vi "pdtV4Main.vi"() -> ()   [LabVIEW 2021]
uses:
  <vilib>/DAQmx/read.llb/DAQmx Read (Analog 1D DBL NChan 1Samp).vi
  <vilib>/DAQmx/create/channels.llb/DAQmx Create Channel (AI-Voltage-Basic).vi
  <vilib>/DAQmx/configure/timing.llb/DAQmx Timing (Sample Clock).vi
  <vilib>/Utility/file.llb/Read Delimited Spreadsheet (DBL).vi
  <vilib>/DAQmx/miscellaneous.llb/DAQmx Fill In Error Info.vi
panel:
  in  "Test time / ms":u32=10000
  out "Pitch y":dbl
  in  "Emergency Stop":bool
  in  "Idle pos":bool
  out "Pitch x":dbl
  in  "Group\nQuantity Y":i32=1
  in  "Group\nQuantity X":i32=1
  out "Initial Y":dbl
  out "Initnal X":dbl
  in  "ConfirmCrd":bool
  out "Instruction":string
  in  "New plate":bool
  in  "Timed Run":bool
  in  "Fine Adjust":bool
  in  "Crd Zero":bool
  out "y":dbl
  out "x":dbl
  in  "Right":bool
  in  "Down":bool
  in  "Left":bool
  in  "Up":bool
  in  "pwm level / 20":i32
  in  "Power Calibration / mW":dbl
  in  "Manual Coordinate Adjustment":bool
  in  "Start PDT":bool
  in  "Plate type":i32(ring) items=["single cell", "96-well 3x3", "96-well 3x2 (horizontal)", "96-well 2x3 (vertical)", "96-well ULA 3x3", "96-well ULA LND 3x2", "24-well 2x2", "96-well flat bottom 3x3 good one"]
  in  "Plate dose / J cm2":dbl[][](array[numeric])
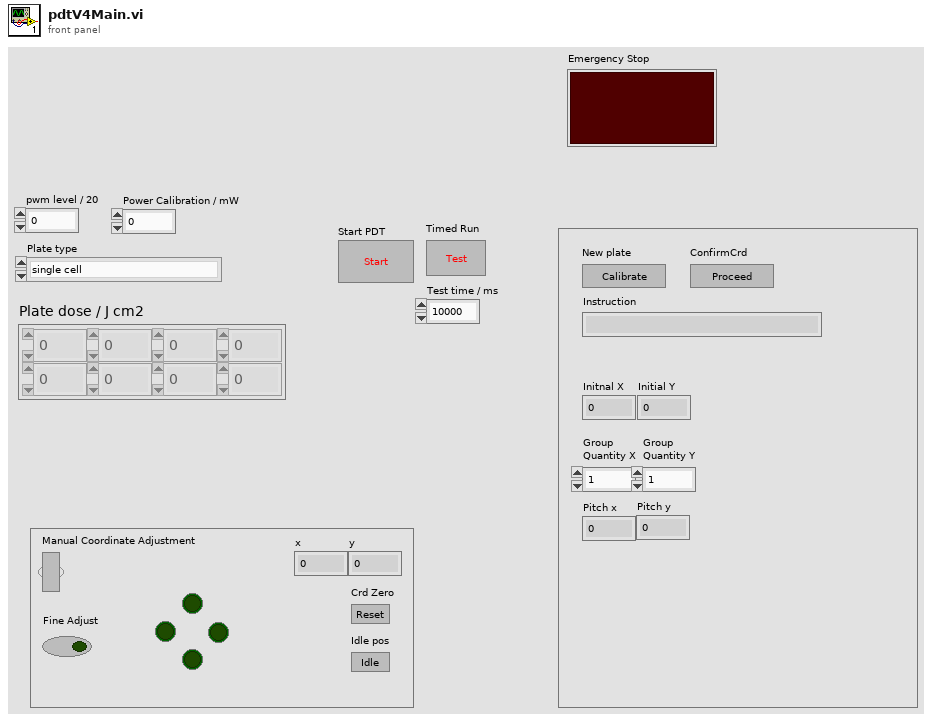
[diagram p1: front panel]
types:
  T1 = enum8{"Enabled", "Disabled", "Disabled and Grayed Out"}
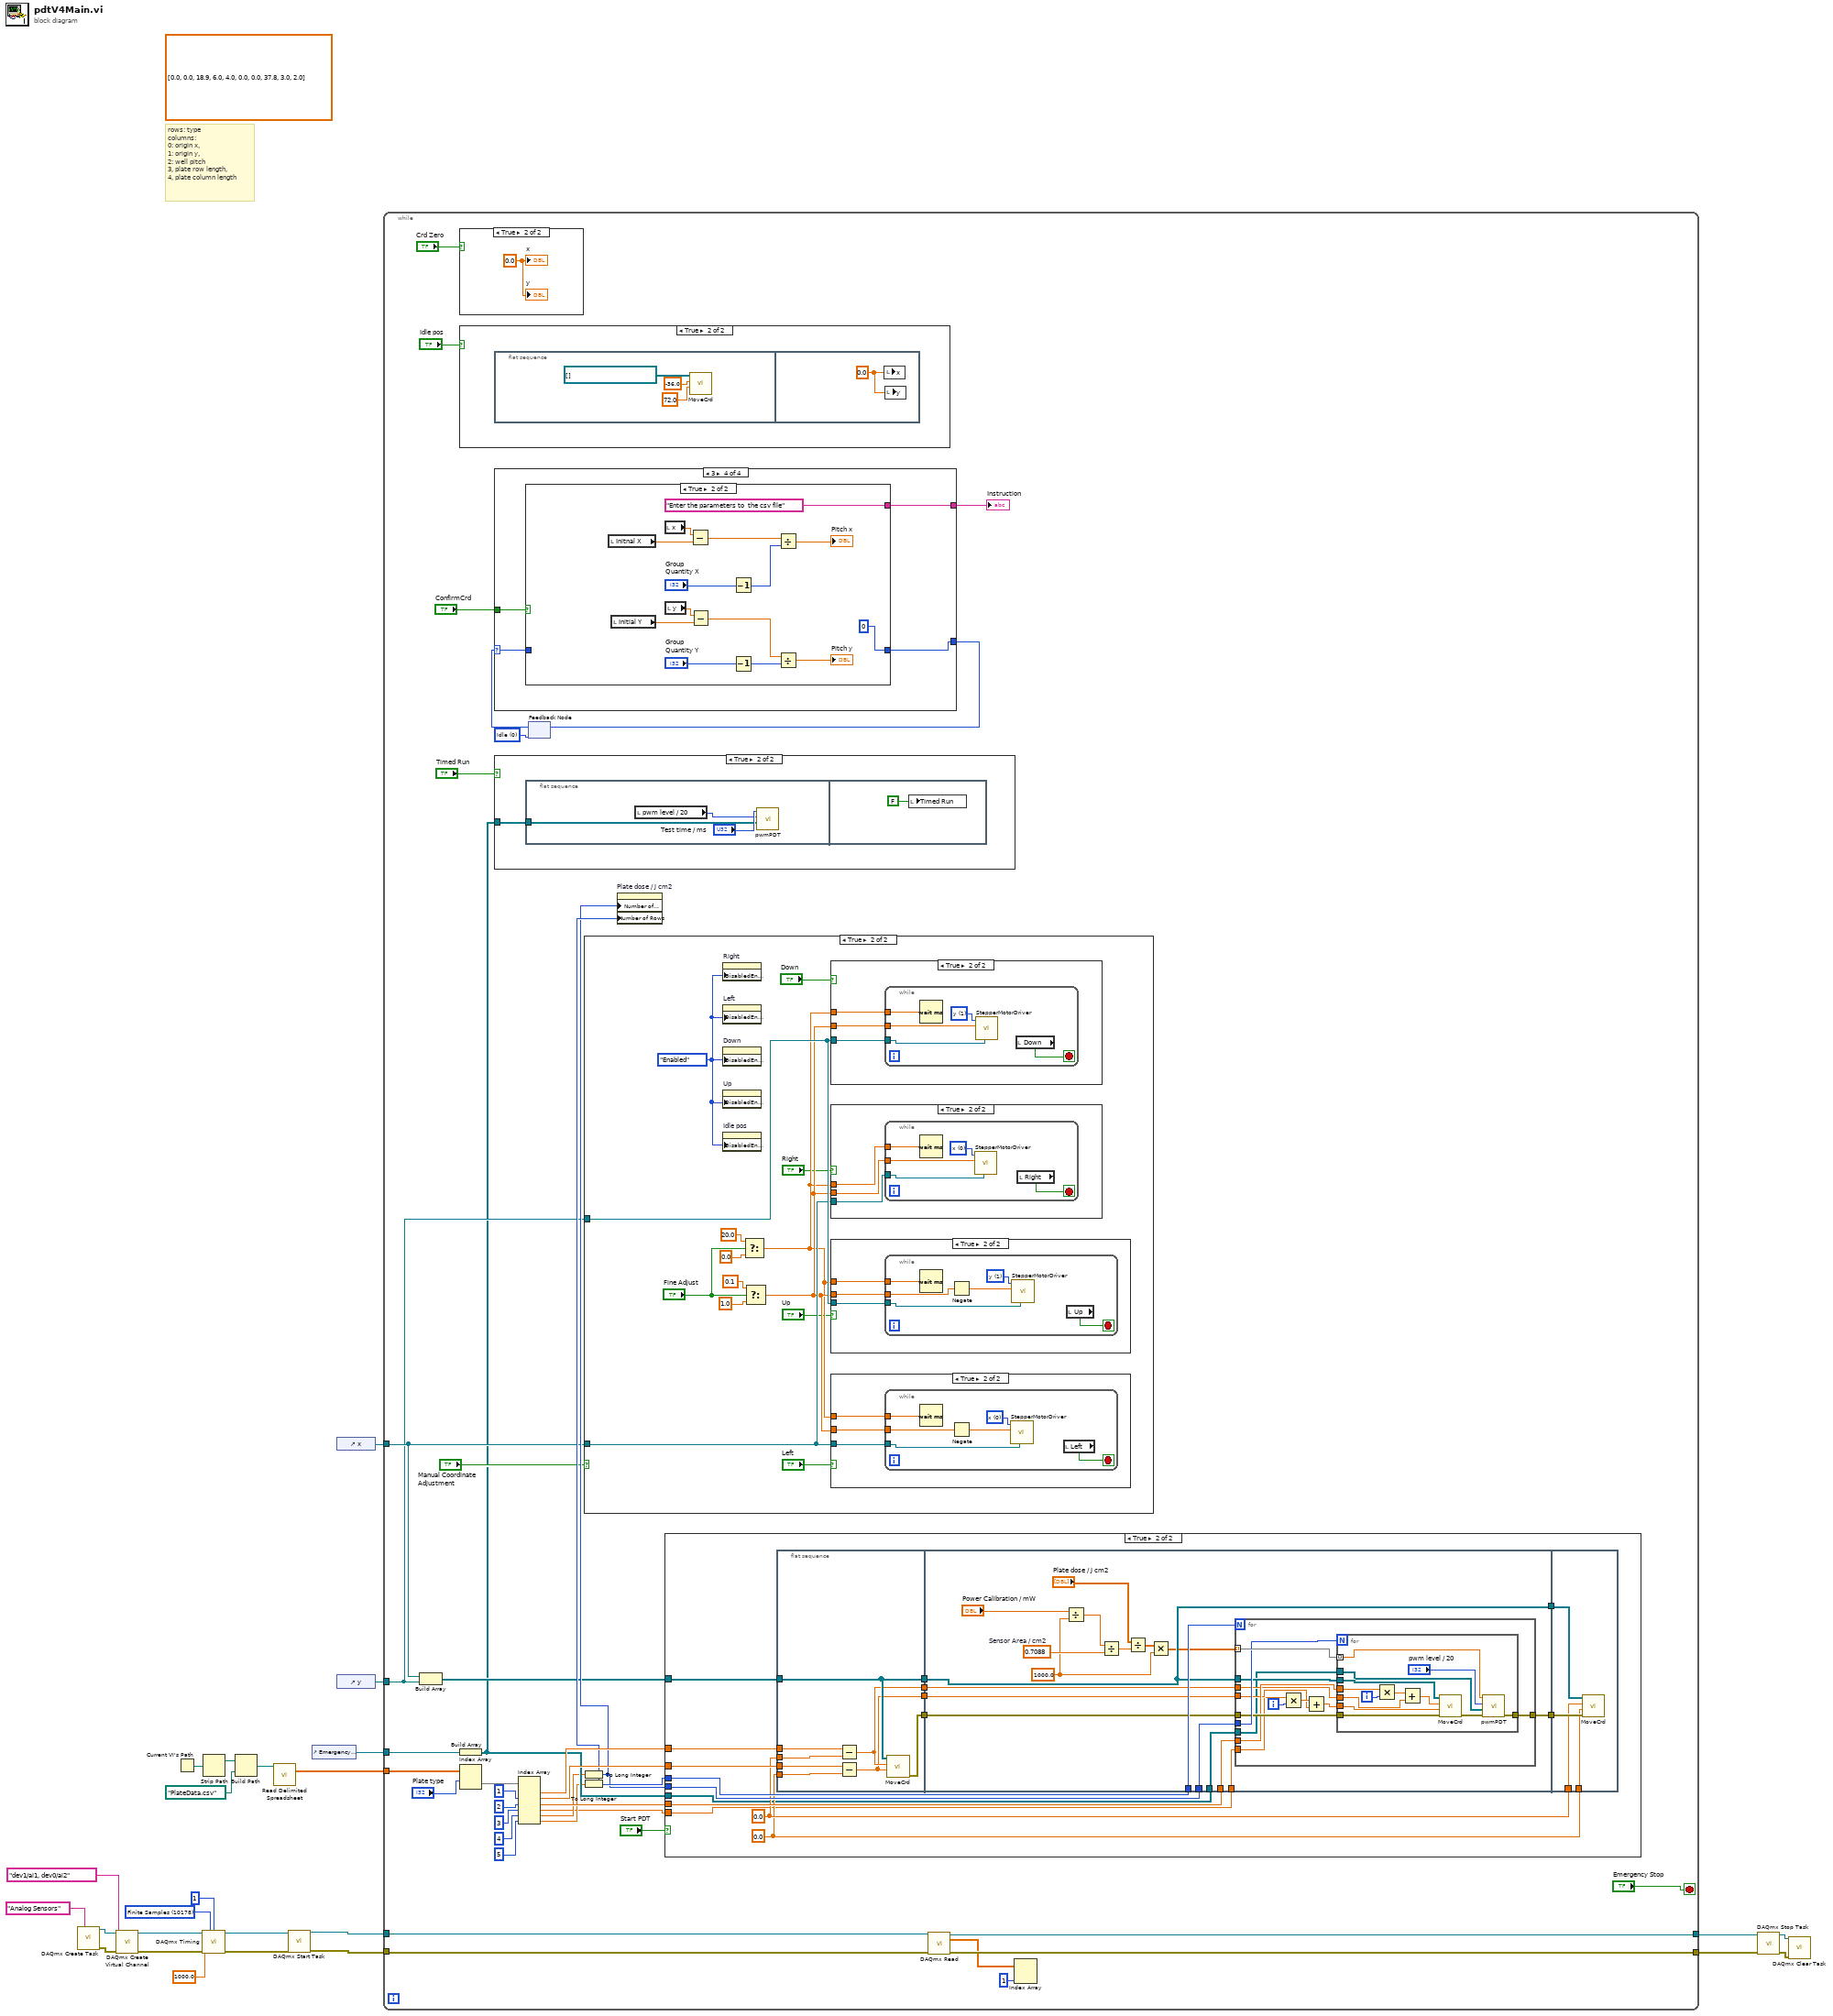
[diagram p0: block diagram]
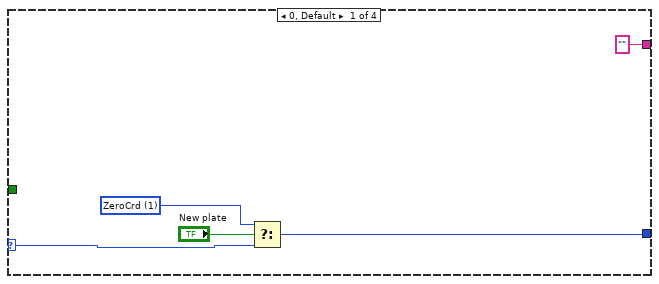
[diagram p3: hidden frame]
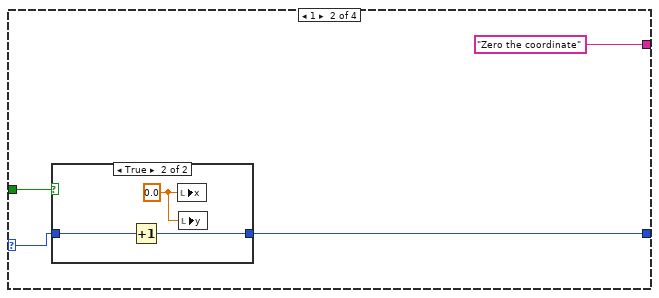
[diagram p4: hidden frame]
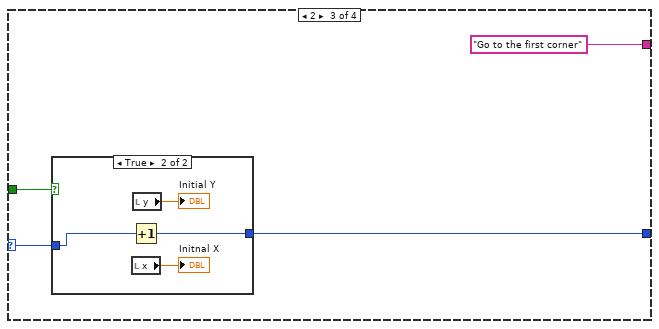
[diagram p6: hidden frame]
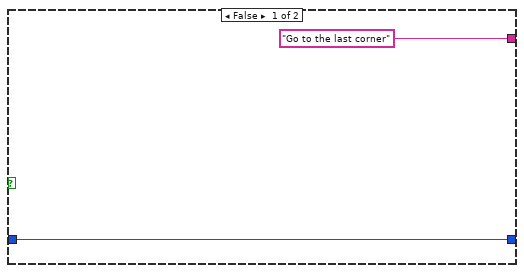
[diagram p8: hidden frame]
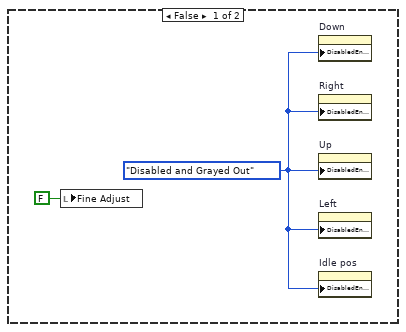
[diagram p11: hidden frame]
diagram:
  w3 = 10178 items=["Finite Samples"=10178, "Continuous Samples"=10123, "Hardware Timed Single Point"=12522] ("sample mode")
  (unwired) dbl[][] [[0.0, 0.0, 18.9, 6.0, 4.0], [0.0, 0.0, 37.8, 3.0, 2.0]]
  # "rows: type\ncolumns: \n0: origin x, \n1: origin y, \n2: well pitch\n3, plate row length, \n4, plate column length"
  n1 = call <vilib>:"DAQmx Create Task.vi"("new task name"="Analog Sensors") -> ("task out"=w7:refnum<k21>, "error out"=w6:errorcluster)  [unwired: 13 in]
  n2 = call-poly <vilib>:"DAQmx Create Virtual Channel.vi"("task in"=w7, "physical channels"=tag "dev1/ai1, dev0/ai2", "error in"=w6) -> ("task out"=w17:refnum<k21>, "error out"=w16:errorcluster)  [unwired: 11 in]
  n3 = Current VI's Path() -> (path=w22:path)
  n4 = call-poly <vilib>:"DAQmx Timing.vi"("task/channels in"=w17, "sample mode"=w3, "samples per channel"=1, "rate"=1000.0, "error in"=w16) -> ("task out"=w15:refnum<k21>, "error out"=w14:errorcluster)  [unwired: 9 in]
  n5 = Strip Path(path=w22) -> (stripped path=w21:path)  [unwired: 1 out]
  n6 = Build Path(base path=w21, name or relative path=path "PlateData.csv" ("file path (dialog if empty)")) -> (appended path=w24:path)
  n7 = call-poly <vilib>:"Read Delimited Spreadsheet.vi"("file path (dialog if empty)"=w24) -> ("all rows"=w25:dbl[][])  [unwired: 9 in, 5 out]
  n8 = call <vilib>:"DAQmx Start Task.vi"("task/channels in"=w15, "error in"=w14) -> ("task out"=w13:refnum<k21>, "error out"=w12:errorcluster)  [unwired: 12 in]
  n9 = control-ref of="Emergency Stop"() -> (w18:refnum<vi>)
  n10 = control-ref of="x"() -> (w20:refnum<vi>)
  n11 = control-ref of="y"() -> (w19:refnum<vi>)
  n12 = while {
    tunnel: w25 -> [w59]
    tunnel: w20 -> [w48]
    tunnel: w19 -> [w40]
    tunnel: w18 -> [w37]
    tunnel: w13 -> [w31]
    tunnel: w12 -> [w30]
    tunnel: [w29] -> w11
    tunnel: [w28] -> w10
    stop <- "Emergency Stop" stop-if-true
    w44 = u16 0 items=["Idle", "ZeroCrd", "StartCorner", "EndCorner"]
    n13 = Build Array(w48, w40) -> (w49:refnum<vi>[])
    n14 = case shown="True" "Crd Zero" {
      frame False {
      }
      frame True {
        w115 = 0.0 ("x")
        "x" <- w115
        "y" <- w115
      }
    }
    n15 = case shown="True" "Idle pos" {
      frame False {
      }
      frame True {
        n16 = flat-sequence {
          frame #0 {
            n17 = call "MoveCrd.vi"("FinalY"=72.0, "FinalX"=-36.0, "Current Crd"=refnum<vi>[] []) -> ()  [unwired: 8 in, 1 out]
          }
          frame #1 {
            w67 = 0.0
            n18 = local write "x"(w67) -> ()
            n19 = local write "y"(w67) -> ()
          }
        }
      }
    }
    n20 = Build Array(w37) -> (w36:refnum<vi>[])
    n21 = Index Array(array=w59, index (row)="Plate type") -> (element=w63:dbl[])  [unwired: 1 in]
    n22 = case shown="True" "Timed Run" {
      tunnel: w36 -> [_ w110]
      frame False {
      }
      frame True {
        n23 = flat-sequence {
          tunnel: w110 -> [w111]
          frame #0 {
            n24 = local read "pwm level / 20"() -> (w112:i32)
            n25 = call "pwmPDT.vi"("EmergencyStop"=w111, "pwm level / 20"=w112, "SetTime / ms"="Test time / ms") -> ()  [unwired: 8 in, 1 out]
          }
          frame #1 {
            n26 = local write "Timed Run"(FALSE ("10 sec pwm")) -> ()
          }
        }
      }
    }
    n27 = Index Array(array=w63, index #2=1 ("index"), index #3=2 ("index"), index #4=3 ("index"), index #5=4 ("index"), index #6=5 ("index")) -> (element #1=w55:dbl, element #2=w54:dbl, element #3=w51:dbl, element #4=w32:dbl, element #5=w33:dbl, element #6=w34:dbl)  [unwired: 1 in]
    n28 = feedback #1(w44) -> (w45:u16)
    n29 = case shown="3" w45 {
      selector: w45 -> [w69 w75 w81 w91]
      tunnel: [w71 w74 w82 w92] -> w43
      tunnel: "ConfirmCrd" -> [_ w76 w83 w93]
      tunnel: ["" ("String") "Zero the coordinate" ("String") "Go to the first corner" ("String") w90] -> w41
      frame 0, Default {
        w72 = u16 1 items=["Idle", "ZeroCrd", "StartCorner", "EndCorner"]
        n30 = Select(t=w72, s="New plate", f=w69) -> (s? t:f=w71:u16)
      }
      frame 1 {
        n31 = case shown="True" w76 {
          tunnel: w75 -> [w77 w79]
          tunnel: [w77 w78] -> w74
          frame False {
          }
          frame True {
            w80 = 0.0
            n32 = Increment(x=w79) -> (x+1=w78:u16)
            n33 = local write "x"(w80) -> ()
            n34 = local write "y"(w80) -> ()
          }
        }
      }
      frame 2 {
        n35 = case shown="True" w83 {
          tunnel: w81 -> [w85 w89]
          tunnel: [w85 w88] -> w82
          frame False {
          }
          frame True {
            n36 = Increment(x=w89) -> (x+1=w88:u16)
            n37 = local read "x"() -> (→"Initnal X":dbl)
            n38 = local read "y"() -> (→"Initial Y":dbl)
          }
        }
      }
      frame 3 {
        n39 = case shown="True" w93 {
          tunnel: [w95 u16 0] -> w92
          tunnel: w91 -> [w95 _]
          tunnel: ["Go to the last corner" ("String") "Enter the parameters to  the csv file" ("String")] -> w90
          frame False {
          }
          frame True {
            n40 = local read "Initnal X"() -> (w108:dbl)
            n41 = local read "Initial Y"() -> (w105:dbl)
            n42 = local read "x"() -> (w109:dbl)
            n43 = local read "y"() -> (w106:dbl)
            n44 = Subtract(x=w109, y=w108) -> (x-y=w107:dbl)
            n45 = Subtract(x=w106, y=w105) -> (x-y=w104:dbl)
            n46 = Decrement(x="Group\nQuantity X") -> (x-1=w101:i32)
            n47 = Decrement(x="Group\nQuantity Y") -> (x-1=w99:i32)
            n48 = Divide(x=w107, y=w101) -> (x/y=→"Pitch x":dbl)
            n49 = Divide(x=w104, y=w99) -> (x/y=→"Pitch y":dbl)
          }
        }
      }
    }
    "Instruction" <- w41
    n50 = feedback-in #1(w43) -> ()
    n51 = To Long Integer(number=w33) -> (32bit integer=w52:i32)
    n52 = To Long Integer(number=w34) -> (32bit integer=w53:i32)
    n53 = case shown="True" "Manual Coordinate Adjustment" {
      tunnel: w40 -> [_ w131]
      tunnel: w48 -> [_ w130]
      frame False {
        w116 = T1."Disabled and Grayed Out" ("Disabled")
        n54 = local write "Fine Adjust"(FALSE ("Fine Adjust")) -> ()
        n55 = property on="Down" class="Bool (strict)"("DisabledEnum"=w116) -> ()  [unwired: 2 in, 2 out]
        n56 = property on="Right" class="Bool (strict)"("DisabledEnum"=w116) -> ()  [unwired: 2 in, 2 out]
        n57 = property on="Up" class="Bool (strict)"("DisabledEnum"=w116) -> ()  [unwired: 2 in, 2 out]
        n58 = property on="Left" class="Bool (strict)"("DisabledEnum"=w116) -> ()  [unwired: 2 in, 2 out]
        n59 = property on="Idle pos" class="Bool"("DisabledEnum"=w116) -> ()  [unwired: 2 in, 2 out]
      }
      frame True {
        w118 = T1."Enabled" ("Disabled")
        n60 = property on="Right" class="Bool (strict)"("DisabledEnum"=w118) -> ()  [unwired: 2 in, 2 out]
        n61 = property on="Left" class="Bool (strict)"("DisabledEnum"=w118) -> ()  [unwired: 2 in, 2 out]
        n62 = property on="Down" class="Bool (strict)"("DisabledEnum"=w118) -> ()  [unwired: 2 in, 2 out]
        n63 = property on="Up" class="Bool (strict)"("DisabledEnum"=w118) -> ()  [unwired: 2 in, 2 out]
        n64 = property on="Idle pos" class="Bool"("DisabledEnum"=w118) -> ()  [unwired: 2 in, 2 out]
        n65 = Select(t=20.0, s="Fine Adjust", f=0.0) -> (s? t:f=w123:dbl)
        n66 = Select(t=0.1, s="Fine Adjust", f=1.0) -> (s? t:f=w127:dbl)
        n67 = case shown="True" "Down" {
          tunnel: w131 -> [_ w134]
          tunnel: w127 -> [_ w133]
          tunnel: w123 -> [_ w132]
          frame False {
          }
          frame True {
            n68 = while {
              tunnel: w134 -> [w137]
              tunnel: w133 -> [w136]
              tunnel: w132 -> [w135]
              stop <- w138 stop-if-true
              w139 = u16 1 items=["x", "y"] ("Direction")
              n69 = Wait (ms)(milliseconds to wait=w135) -> ()  [unwired: 1 out]
              n70 = call "StepperMotorDriver.vi"("pCoordinate"=w137, "Distance"=w136, "Direction"=w139) -> ()  [unwired: 8 in, 1 out]
              n71 = local read "Down"() -> (w138:bool)
            }
          }
        }
        n72 = case shown="True" "Right" {
          tunnel: w130 -> [_ w151]
          tunnel: w127 -> [_ w150]
          tunnel: w123 -> [_ w149]
          frame False {
          }
          frame True {
            n73 = while {
              tunnel: w151 -> [w154]
              tunnel: w150 -> [w153]
              tunnel: w149 -> [w152]
              stop <- w155 stop-if-true
              w156 = u16 0 items=["x", "y"] ("Direction")
              n74 = Wait (ms)(milliseconds to wait=w152) -> ()  [unwired: 1 out]
              n75 = call "StepperMotorDriver.vi"("pCoordinate"=w154, "Distance"=w153, "Direction"=w156) -> ()  [unwired: 8 in, 1 out]
              n76 = local read "Right"() -> (w155:bool)
            }
          }
        }
        n77 = case shown="True" "Up" {
          tunnel: w131 -> [_ w159]
          tunnel: w127 -> [_ w158]
          tunnel: w123 -> [_ w157]
          frame False {
          }
          frame True {
            n78 = while {
              tunnel: w159 -> [w163]
              tunnel: w158 -> [w162]
              tunnel: w157 -> [w160]
              stop <- w164 stop-if-true
              w165 = u16 1 items=["x", "y"] ("Direction")
              n79 = Wait (ms)(milliseconds to wait=w160) -> ()  [unwired: 1 out]
              n80 = Negate(x=w162) -> (-x=w161:dbl)
              n81 = call "StepperMotorDriver.vi"("pCoordinate"=w163, "Distance"=w161, "Direction"=w165) -> ()  [unwired: 8 in, 1 out]
              n82 = local read "Up"() -> (w164:bool)
            }
          }
        }
        n83 = case shown="True" "Left" {
          tunnel: w130 -> [_ w142]
          tunnel: w127 -> [_ w141]
          tunnel: w123 -> [_ w140]
          frame False {
          }
          frame True {
            n84 = while {
              tunnel: w142 -> [w146]
              tunnel: w141 -> [w145]
              tunnel: w140 -> [w143]
              stop <- w147 stop-if-true
              w148 = u16 0 items=["x", "y"] ("Direction")
              n85 = Wait (ms)(milliseconds to wait=w143) -> ()  [unwired: 1 out]
              n86 = Negate(x=w145) -> (-x=w144:dbl)
              n87 = call "StepperMotorDriver.vi"("pCoordinate"=w146, "Distance"=w144, "Direction"=w148) -> ()  [unwired: 8 in, 1 out]
              n88 = local read "Left"() -> (w147:bool)
            }
          }
        }
      }
    }
    n89 = property on="Plate dose / J cm2" class="Arr (strict)"("Number of Columns"=w52, "Number of Rows"=w53) -> ()  [unwired: 2 in, 2 out]
    n90 = case shown="True" "Start PDT" {
      tunnel: w55 -> [_ w179]
      tunnel: w54 -> [_ w181]
      tunnel: w53 -> [_ w178]
      tunnel: w52 -> [_ w180]
      tunnel: w51 -> [_ w174]
      tunnel: w49 -> [_ w177]
      tunnel: w36 -> [_ w167]
      tunnel: w32 -> [_ w166]
      frame False {
      }
      frame True {
        w171 = 0.0 ("y")
        w170 = 0.0 ("y")
        n91 = flat-sequence {
          tunnel: w179 -> [w189]
          tunnel: w181 -> [w188]
          tunnel: w177 -> [w186]
          tunnel: [w187] -> w176
          tunnel: [w186] -> w175
          tunnel: w170 -> [w185]
          tunnel: w171 -> [w184]
          tunnel: [w182] -> w169
          tunnel: [w183] -> w168
          tunnel: w178 -> [w207]
          tunnel: w180 -> [w206]
          tunnel: w176 -> [w203]
          tunnel: w175 -> [w200]
          tunnel: w174 -> [w202]
          tunnel: [w201] -> w173
          tunnel: [w200] -> w172
          tunnel: w169 -> [w193]
          tunnel: w168 -> [w192]
          tunnel: w167 -> [w191]
          tunnel: w166 -> [w190]
          tunnel: w173 -> [w237]
          tunnel: w172 -> [w236]
          tunnel: w171 -> [w235]
          tunnel: w170 -> [w234]
          frame #0 {
            n92 = Subtract(x=w189, y=w184) -> (x-y=w183:dbl)
            n93 = Subtract(x=w188, y=w185) -> (x-y=w182:dbl)
            n94 = call "MoveCrd.vi"("FinalY"=w182, "FinalX"=w183, "Current Crd"=w186) -> ("error out"=w187:errorcluster)  [unwired: 8 in]
          }
          frame #1 {
            w199 = 0.7088  # Sensor Area / cm2
            w194 = 1000.0 ("y")
            n95 = Divide(x="Power Calibration / mW", y=w194) -> (x/y=w197:dbl)
            n96 = Divide(x=w197, y=w199) -> (x/y=w204:dbl)
            n97 = Divide(x="Plate dose / J cm2", y=w204) -> (x/y=w196:dbl[][])
            n98 = Multiply(x=w196, y=w194) -> (x*y=w195:dbl[][])
            n99 = for {
              N: w207 -> [_]
              tunnel: w206 -> [w219]
              tunnel: w195 -> [w220] mode=indexing
              tunnel: w203 -> [w218]
              tunnel: w200 -> [w217]
              tunnel: w202 -> [w215]
              tunnel: [w214] -> w201
              tunnel: w193 -> [w211]
              tunnel: w192 -> [w210]
              tunnel: w191 -> [w209]
              tunnel: w190 -> [w208]
              i -> [w216]
              n100 = Multiply(x=w208, y=w216) -> (x*y=w213:dbl)
              n101 = Add(x=w213, y=w211) -> (x+y=w212:dbl)
              n102 = for {
                N: w219 -> [_]
                tunnel: w220 -> [w232] mode=indexing
                tunnel: [w231] -> w214
                tunnel: w218 -> [w230]
                tunnel: w217 -> [w229]
                tunnel: w215 -> [w226]
                tunnel: w212 -> [w225]
                tunnel: w210 -> [w222]
                tunnel: w209 -> [w221]
                i -> [w227]
                n103 = Multiply(x=w226, y=w227) -> (x*y=w224:dbl)
                n104 = Add(x=w224, y=w222) -> (x+y=w223:dbl)
                n105 = call "MoveCrd.vi"("error in"=w230, "FinalY"=w225, "FinalX"=w223, "Current Crd"=w229) -> ("error out"=w228:errorcluster)  [unwired: 7 in]
                n106 = call "pwmPDT.vi"("error in"=w228, "EmergencyStop"=w221, "pwm level / 20"="pwm level / 20", "SetTime / ms"=w232) -> ("error out"=w231:errorcluster)  [unwired: 7 in]
              }
            }
          }
          frame #2 {
            n107 = call "MoveCrd.vi"("error in"=w237, "FinalY"=w234, "FinalX"=w235, "Current Crd"=w236) -> ()  [unwired: 7 in, 1 out]
          }
        }
      }
    }
    n108 = call-poly <vilib>:"DAQmx Read.vi"("task/channels in"=w31, "error in"=w30) -> ("task out"=w29:refnum<k21>, "data"=w27:dbl[], "error out"=w28:errorcluster)  [unwired: 11 in]
    n109 = Index Array(array=w27, index #2=1 ("index")) -> ()  [unwired: 1 in, 2 out]
  }
  n110 = call <vilib>:"DAQmx Stop Task.vi"("task/channels in"=w11, "error in"=w10) -> ("task out"=w9:refnum<k21>, "error out"=w8:errorcluster)  [unwired: 12 in]
  n111 = call <vilib>:"DAQmx Clear Task.vi"("task in"=w9, "error in"=w8) -> ()  [unwired: 13 in, 1 out]
